vi "Init.vi"(8 "error in (no error)":errorcluster, 11 "CloneRegRef":refnum<data-value>) -> (0 "error out":errorcluster, 3 "CloneRegRef":refnum<data-value>)   [LabVIEW 2018, in "ModuleAdmin.lvlib" / "CloneRegistration.lvclass"]
uses:
  CloneRegistration.lvclass
  CloneRegistration.lvclass/CloneRegistration.ctl
  Accessors/Write vRegistry.vi
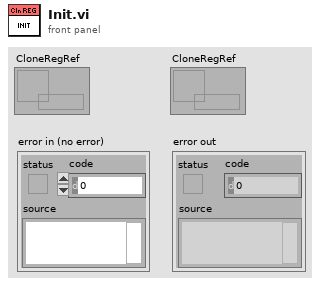
[diagram p1: front panel]
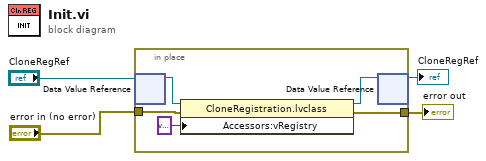
[diagram p0: block diagram]
diagram:
  n1 = in-place {
    in-place-border: "error in (no error)" -> [w6]
    in-place-border: [w5] -> w1
    n2 = in-place-dvr #1("CloneRegRef") -> (w8:refnum<class "CloneRegistration.lvclass">)  [unwired: 1 out]
    n3 = property class="CloneRegistration.lvclass"(reference=w8, error in=w6, "Accessors:vRegistry"=variant ("vRegistry")) -> (reference out=w7:refnum<class "CloneRegistration.lvclass">, error out=w5:errorcluster)
    n4 = in-place-dvr #1(w7) -> (→"CloneRegRef":refnum<data-value>)  [unwired: 1 out]
  }
  "error out" <- w1
